vi "Graph-to-2D-SVG.vi"(10 "file path (use dialog)":path=path "C:/Users/Phil/Desktop/SVGTest.html", 11 "Conductance":T1(array[cluster])) -> (3 "HTML SVG":string)   [LabVIEW 2016]
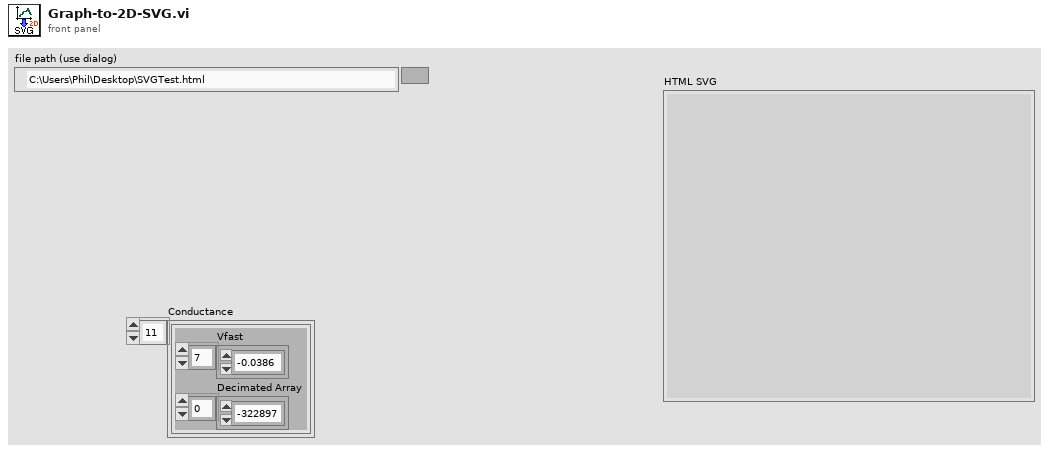
[diagram p1: front panel]
types:
  T1 = cluster{"Vfast":dbl[], "Decimated Array":dbl[]}[]
  T2 = enum16{"open", "replace", "create", "open or create", "replace or create", "replace or create with confirmation"}
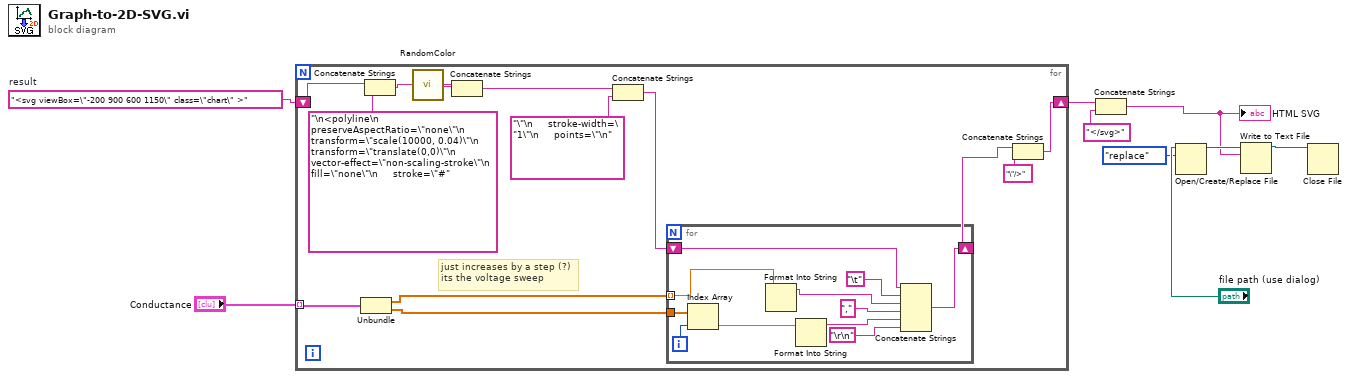
[diagram p0: block diagram]
diagram:
  w8 = "<svg viewBox=\"-200 900 600 1150\" class=\"chart\" >"  # result
  n1 = for {
    tunnel: "Conductance" -> [w22] mode=indexing
    shift-right: [w17] -> w7
    shift-left: w8 -> [w19]
    # "just increases by a step (?)\nits the voltage sweep"
    n2 = Unbundle(w22) -> ("Vfast"=w21:dbl[], "Decimated Array"=w20:dbl[])
    n3 = Concatenate Strings(w19, "\n<polyline\n     preserveAspectRatio=\"none\"\n     transform=\"scale(10000, 0.04)\"\n     transform=\"translate(0,0)\"\n     vector-effect=\"non-scaling-stroke\"\n     fill=\"none\"\n     stroke=\"#") -> (w11:string)
    n4 = call "RandomColor.vi"() -> ("String"=w12:string)  [unwired: 11 in]
    n5 = Concatenate Strings(w11, w12) -> (w10:string)
    n6 = Concatenate Strings(w10, "\"\n     stroke-width=\"1\"\n     points=\"\n") -> (w13:string)
    n7 = for {
      tunnel: w21 -> [w31] mode=indexing
      tunnel: w20 -> [w33]
      shift-right: [w29] -> w15
      shift-left: w13 -> [w28]
      i -> [w32]
      n8 = Index Array(array=w33, index=w32) -> (element=w30:dbl)
      n9 = Format Into String(w31) -> (resulting string=w24:string)  [unwired: 3 in, 1 out]
      n10 = Format Into String(w30) -> (resulting string=w26:string)  [unwired: 3 in, 1 out]
      n11 = Concatenate Strings(w28, "\t", w24, ",", w26, "\r\n") -> (w29:string)
    }
    n12 = Concatenate Strings(w15, "\"/>") -> (w17:string)
  }
  n13 = Concatenate Strings(w7, "</svg>") -> (w4:string)
  "HTML SVG" <- w4
  n14 = Open/Create/Replace File(file path (use dialog)="file path (use dialog)", operation (0:open)=T2."replace") -> (refnum out=w5:refnum<file>)  [unwired: 4 in, 2 out]
  n15 = Write to Text File(file (use dialog)=w5, text=w4) -> (refnum out=w2:refnum<file>)  [unwired: 2 in, 2 out]
  n16 = Close File(refnum=w2) -> ()  [unwired: 1 in, 2 out]
